vi "MergeError.vi"(8 "error in (no error)":errorcluster, 11 "Error":T1) -> (0 "error out":errorcluster)   [LabVIEW 2020]
uses:
  <vilib>/NI VeriStand/Execution/Workspace/ErrorInfo.ctl
  NationalInstruments.VeriStand
  <vilib>/NI VeriStand/Execution/Workspace/NI_VS Workspace ExecutionAPI.lvlib
panel:
  in  "VeriStand":string="NI VeriStand"
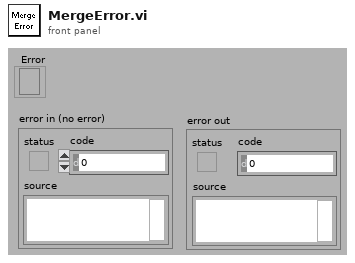
[diagram p1: front panel]
types:
  T1 = typedef "NI_VS Workspace ExecutionAPI.lvlib/ErrorInfo.ctl" = refnum<k24>
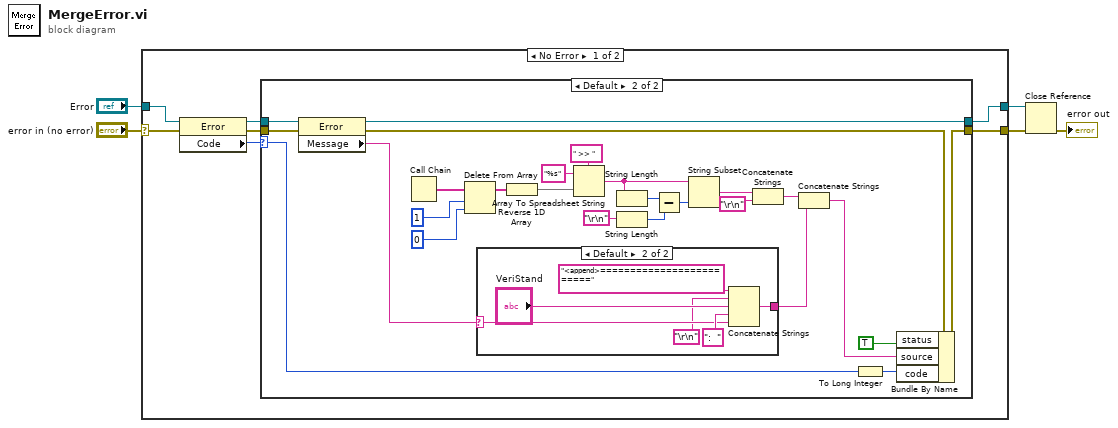
[diagram p0: block diagram]
diagram:
  n1 = case shown="No Error" "error in (no error)" {
    selector: "error in (no error)" -> [w12 w49]
    tunnel: [w10 w49] -> w1
    tunnel: [w6 w48] -> w2
    tunnel: "Error" -> [w9 w48]
    frame No Error {
      n2 = property class="Error"(reference=w9, error in=w12) -> (reference out=w7:T1, error out=w11:errorcluster, "Code"=w8:u32)
      n3 = case shown="Default" w8 {
        selector: w8 -> [_ w16]
        tunnel: [w14 w40] -> w10
        tunnel: w11 -> [w14 w20]
        tunnel: w7 -> [w13 w22]
        tunnel: [w13 w21] -> w6
        frame 0 {
        }
        frame Default {
          n4 = property class="Error"(reference=w22, error in=w20) -> (reference out=w21:T1, error out=w19:errorcluster, "Message"=w18:string)
          n5 = Call Chain() -> (call chain=w31:string[])
          n6 = Delete From Array(array=w31, length=1 ("CallChainLvl"), index=0) -> (array with subset deleted=w27:string[])  [unwired: 1 out]
          n7 = case shown="Default" w18 {
            selector: w18 -> [w41 w44]
            tunnel: [w41 w45] -> w35
            frame "" {
            }
            frame Default {
              n8 = Concatenate Strings("<append>=========================", "\r\n", "VeriStand", ":  " ("string"), w44) -> (w45:string)
            }
          }
          n9 = Reverse 1D Array(array=w27) -> (reversed array=w28:string[])
          n10 = Array To Spreadsheet String(delimiter (Tab)=" >> ", array=w28, 3:"%s" ("format string")) -> (spreadsheet string=w26:string)
          n11 = String Length(string=w26) -> (length=w29:i32)
          n12 = String Length(string="\r\n") -> (length=w24:i32)
          n13 = Subtract(x=w29, y=w24) -> (x-y=w30:i32)
          n14 = String Subset(string=w26, length (rest)=w30) -> (substring=w36:string)  [unwired: 1 out]
          n15 = Concatenate Strings(w36, "\r\n") -> (w37:string)
          n16 = Concatenate Strings(w37, w35) -> (w38:string)
          n17 = To Long Integer(number=w16) -> (32bit integer=w15:i32)
          n18 = Bundle By Name(cluster=w19, "status"=TRUE, "source"=w38, "code"=w15) -> (w40:errorcluster)
        }
      }
    }
    frame Error {
      # "Cluster already contains error"
    }
  }
  n19 = Close Reference(reference=w2, error in (no error)=w1) -> (error out=→"error out":errorcluster)
